vi "Calculate Checksum.vi"(1 "String in":string) -> (0 "Checksum":u16 format="%.0x")   [LabVIEW 2014, in "KIT QV.lvlib"]
doc: "Compute checksum as 4-digit HEX string and append to String in."
uses:
  KIT QV.lvlib
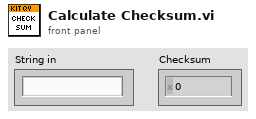
[diagram p1: front panel]
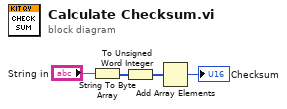
[diagram p0: block diagram]
diagram:
  n1 = String To Byte Array(string="String in") -> (unsigned byte array=w3:u8[])
  n2 = To Unsigned Word Integer(number=w3) -> (unsigned 16bit integer=w2:u16[])
  n3 = Add Array Elements(numeric array=w2) -> (sum=→"Checksum":u16)
